vi "Key - Cluster Read.vi"(8 "error in (no error)":errorcluster, 9 "New Ctl Ref":refnum<vi>, 10 "Original Ctl Ref":refnum<vi>, 11 "Refnum in":T1) -> (0 "error out":errorcluster, 2 "spreadsheet string":string[](array[string]), 3 "Refnum out":T1)   [LabVIEW 2013]
uses:
  <vilib>/Utility/config.llb/Config Data RefNum.ctl
  <vilib>/Utility/config.llb/Read Key (String).vi
  <vilib>/Utility/config.llb/NI_LVConfig.lvlib
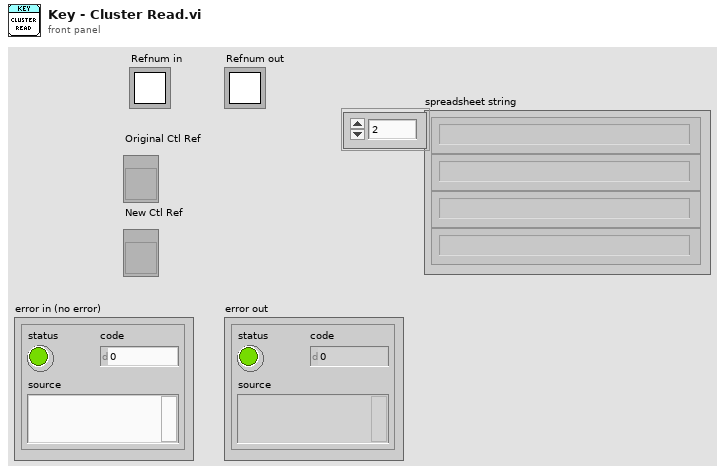
[diagram p1: front panel]
types:
  T1 = typedef "NI_LVConfig.lvlib/Config Data RefNum.ctl" = refnum<k1>
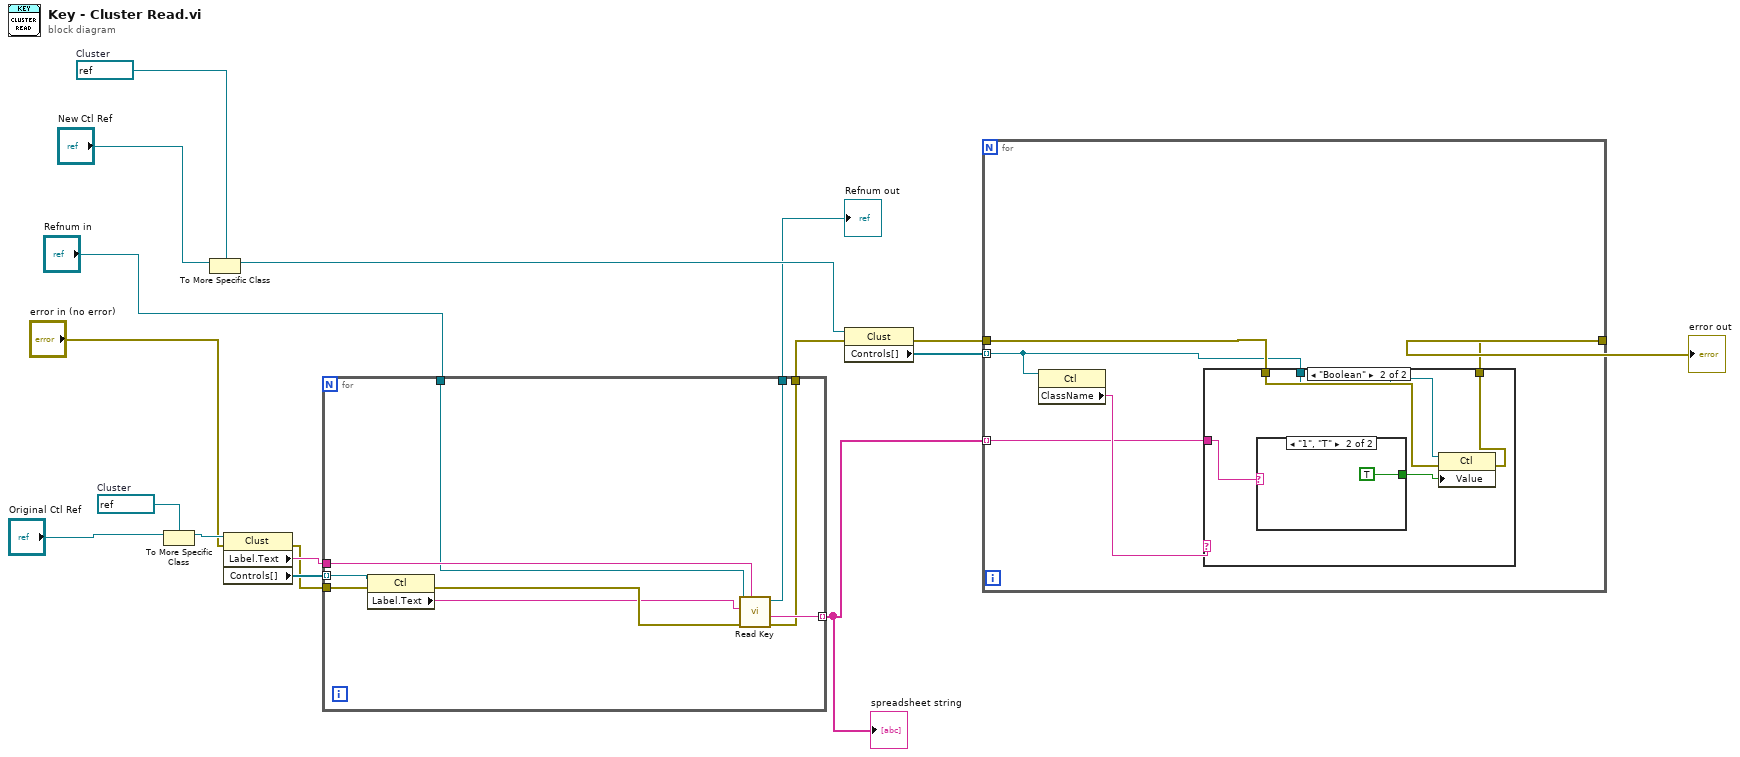
[diagram p0: block diagram]
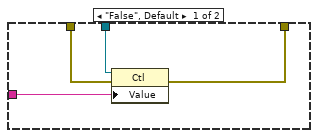
[diagram p2: hidden frame]
diagram:
  w10 = refnum<vi> refnum  # Cluster
  w13 = refnum<vi> refnum  # Cluster
  n1 = To More Specific Class(target class=w10, reference="Original Ctl Ref") -> (specific class reference=w9:refnum<vi>)  [unwired: 1 in, 1 out]
  n2 = To More Specific Class(target class=w13, reference="New Ctl Ref") -> (specific class reference=w12:refnum<vi>)  [unwired: 1 in, 1 out]
  n3 = property class="Clust"(reference=w9, error in="error in (no error)") -> (error out=w2:errorcluster, "Label.Text"=w7:string, "Controls[]"=w8:refnum<vi>[])  [unwired: 1 out]
  n4 = for {
    tunnel: w8 -> [w26] mode=indexing
    tunnel: w7 -> [w25]
    tunnel: "Refnum in" -> [w24]
    tunnel: [w23] -> w1 mode=indexing
    tunnel: [w22] -> w5
    tunnel: [w21] -> w3
    tunnel: w2 -> [w19]
    n5 = property class="Ctl"(reference=w26, error in=w19) -> (error out=w20:errorcluster, "Label.Text"=w18:string)  [unwired: 1 out]
    n6 = call-poly <vilib>:"Read Key.vi"("section"=w25, "error in (no error)"=w20, "key"=w18, "refnum"=w24) -> ("error out"=w21:errorcluster, "value"=w23:string, "refnum out"=w22:T1)  [unwired: 4 in, 1 out]
  }
  "Refnum out" <- w5
  "spreadsheet string" <- w1
  n7 = property class="Clust"(reference=w12, error in=w3) -> (error out=w16:errorcluster, "Controls[]"=w15:refnum<vi>[])  [unwired: 1 out]
  n8 = for {
    tunnel: w15 -> [w29] mode=indexing
    tunnel: w16 -> [w31]
    tunnel: [w30] -> w17
    tunnel: w1 -> [w27] mode=indexing
    n9 = property class="Ctl"(reference=w29) -> ("ClassName"=w28:string)  [unwired: 1 in, 2 out]
    n10 = case shown="\"Boolean\"" w28 {
      tunnel: w27 -> [w35 w36]
      tunnel: w29 -> [w34 w38]
      tunnel: w31 -> [w33 w39]
      tunnel: [w32 w37] -> w30
      frame "False", Default {
        n11 = property class="Ctl"(reference=w34, error in=w33, "Value"=w35) -> (error out=w32:errorcluster)  [unwired: 1 out]
      }
      frame "Boolean" {
        n12 = case shown="\"1\", \"T\"" w36 {
          tunnel: [_ TRUE] -> w40
          frame "False", Default {
          }
          frame "1", "T" {
          }
        }
        n13 = property class="Ctl"(reference=w38, error in=w39, "Value"=w40) -> (error out=w37:errorcluster)  [unwired: 1 out]
      }
    }
  }
  "error out" <- w17
